vi "Pololu.Mgr - Set Channel OFF.vi"(8 "error in (no error)":errorcluster, 10 "Channel":u8, 11 "PololuCtrl in":refnum<class "PololuCtrl.lvclass">) -> (0 "error out":errorcluster, 3 "PololuCtrl out":refnum<class "PololuCtrl.lvclass">)   [LabVIEW 2018, in "PololuCtrl.lvclass"]
uses:
  PololuCtrl.lvclass
  SubVIs/Pololu.Message Byte Defs.ctl
  PololuCtrl.lvclass/PololuCtrl.ctl
  Serial Port/Class/SerialPort.lvclass
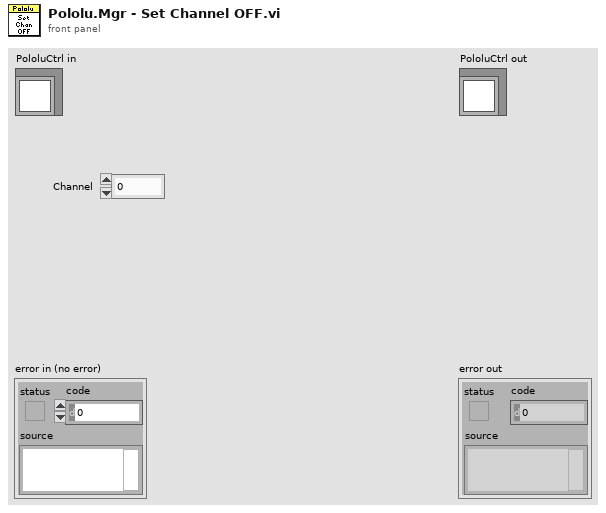
[diagram p1: front panel]
types:
  T1 = cluster{"Channel":u8, "Pos":u16, "Response":u16, "Bytes":u8[], "Query":bool}
  T2 = typedef "Pololu.Message Byte Defs.ctl" = u8
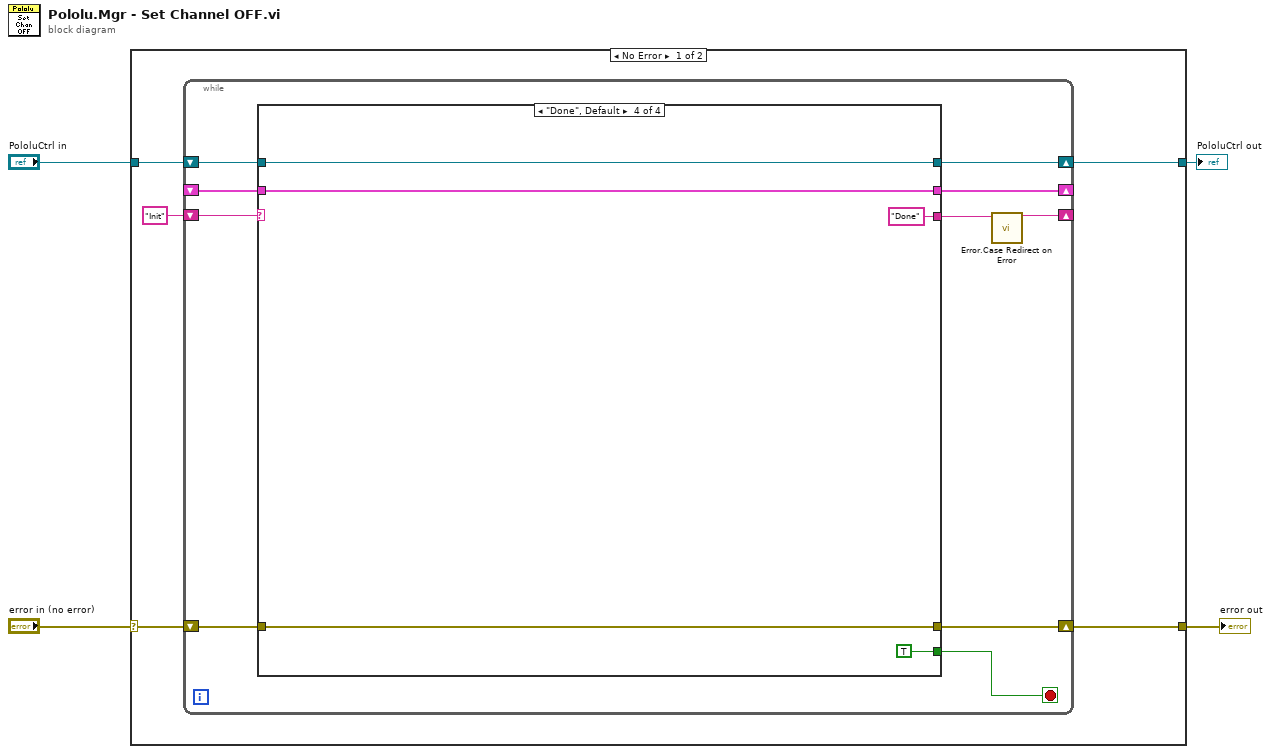
[diagram p0: block diagram]
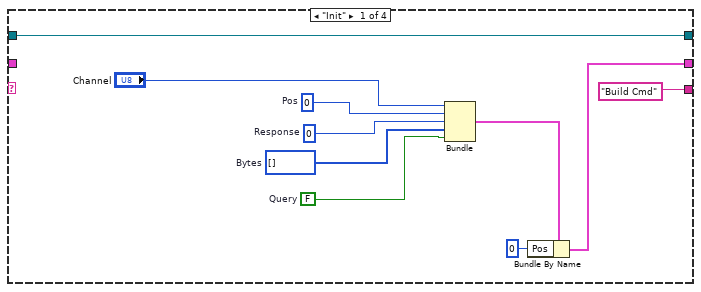
[diagram p2: hidden frame]
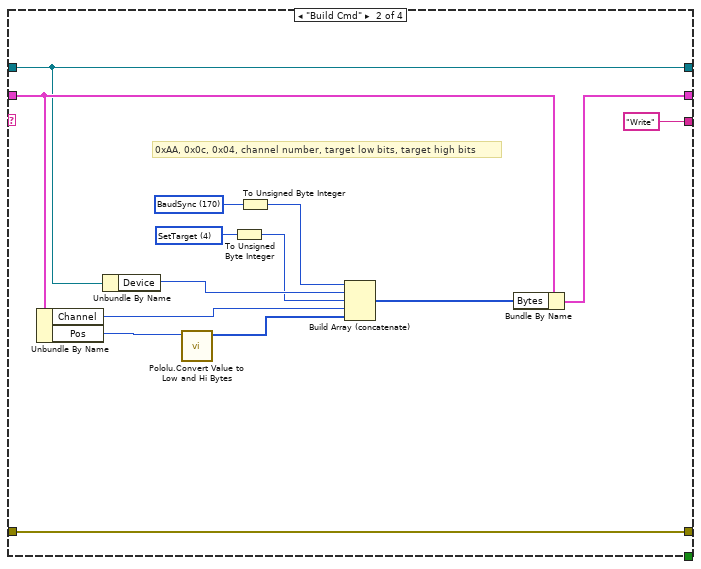
[diagram p3: hidden frame]
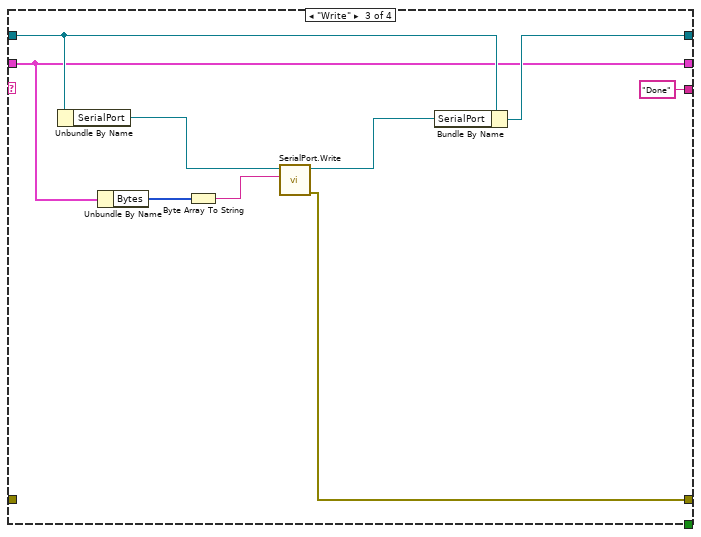
[diagram p4: hidden frame]
diagram:
  n1 = case shown="No Error" "error in (no error)" {
    selector: "error in (no error)" -> [w8 w59]
    tunnel: [w5 w59] -> w3
    tunnel: [w7 w58] -> w1
    tunnel: "PololuCtrl in" -> [w9 w58]
    frame No Error {
      n2 = while {
        shift-right: [w18] -> w7
        shift-left: w9 -> [w19]
        shift-right: [w11] -> w5
        shift-left: w8 -> [w12]
        shift-right: [w15] -> _
        shift-left: "Init" -> [w16]
        shift-right: [w13] -> _
        shift-left: _ -> [w17]
        stop <- w10 stop-if-true
        n3 = case shown="\"Done\", Default" w16 {
          tunnel: w19 -> [w24 w37 w49 w57]
          tunnel: [w24 w37 w50 w57] -> w18
          tunnel: w17 -> [_ w41 w45 w54]
          tunnel: ["Build Cmd" "Write" "Done" "Done"] -> w14
          tunnel: [w22 w42 w45 w54] -> w13
          tunnel: w12 -> [_ w43 _ w55]
          tunnel: [_ w43 w46 w55] -> w11
          tunnel: [_ _ _ TRUE] -> w10
          frame "Init" {
            w25 = u16 0  # Pos
            w28 = u16 0  # Response
            w26 = FALSE  # Query
            w27 = u8[] []  # Bytes
            n4 = Bundle("Channel"="Channel", "Pos"=w25, "Response"=w28, "Bytes"=w27, "Query"=w26) -> (w23:T1)  [unwired: 1 in]
            n5 = Bundle By Name(cluster=w23, "Pos"=u16 0) -> (w22:T1)
          }
          frame "Build Cmd" {
            w31 = T2 4 items=["BaudSync"=170, "SetTarget"=4, "Set Speed"=7, "Set Accel"=9, "Get Pos"=16, "Get MovStat"=19, "Get Errors"=33] ("Cmds")
            w32 = T2 170 items=["BaudSync"=170, "SetTarget"=4, "Set Speed"=7, "Set Accel"=9, "Get Pos"=16, "Get MovStat"=19, "Get Errors"=33] ("Cmds")
            # "0xAA, 0x0c, 0x04, channel number, target low bits, target high bits"
            n6 = Unbundle By Name(w41) -> ("Channel"=w40:u8, "Pos"=w39:u16)
            n7 = Unbundle By Name(w37) -> ("Device"=w36:u8)
            n8 = call "Pololu.Convert Value to Low and Hi Bytes.vi"("Value"=w39) -> ("Low_Hi Bytes"=w33:u8[])  [unwired: 10 in]
            n9 = To Unsigned Byte Integer(number=w31) -> (unsigned 8bit integer=w34:T2)
            n10 = To Unsigned Byte Integer(number=w32) -> (unsigned 8bit integer=w35:T2)
            n11 = Build Array (concatenate)(w35, w36, w34, w40, w33) -> (w38:T2[])
            n12 = Bundle By Name(cluster=w41, "Bytes"=w38) -> (w42:T1)
          }
          frame "Write" {
            n13 = Unbundle By Name(w49) -> ("SerialPort"=w48:refnum<class "SerialPort.lvclass">)
            n14 = Unbundle By Name(w45) -> ("Bytes"=w51:u8[])
            n15 = Byte Array To String(unsigned byte array=w51) -> (string=w44:string)
            n16 = call "SerialPort.Write.vi"("Data"=w44, "SerialPort in"=w48) -> ("error out"=w46:errorcluster, "SerialPort out"=w47:refnum<class "SerialPort.lvclass">)  [unwired: 6 in, 2 out]
            n17 = Bundle By Name(cluster=w49, "SerialPort"=w47) -> (w50:refnum<class "PololuCtrl.lvclass">)
          }
          frame "Done", Default {
          }
        }
        n18 = call "Error.Case Redirect on Error.vi"("Next Case"=w14) -> ("Next Case Out"=w15:string)  [unwired: 10 in]
      }
    }
    frame Error {
    }
  }
  "error out" <- w3
  "PololuCtrl out" <- w1
